vi "GetSetParam.vi"() -> ()   [LabVIEW 2020]
uses:
  lib/Snap7.lvlib
panel:
  out "?":string
  in  "Value":i64=500
  in  "Param to Set":i32(ring)=3 items=["Local Port"=1, "Remote Port"=2, "Ping Timeout (ms)"=3, "Send Timeout (ms)"=4, "Recv Timeout (ms)"=5, "Work Interval (ms)"=6, "Source REF"=7, "Destination REF"=8, "Source TSAP"=9, "PDU Request"=10, "Max Clients"=11, "BSend Timeout (ms)"=12, "BRecv Timeout (ms)"=13, "Recovery Time (ms)"=14, "Keep Alive Time (ms)"=15]
  out "ParamValue":i32
  in  "ParamNumber":i32(ring)=2 items=["Local Port"=1, "Remote Port"=2, "Ping Timeout (ms)"=3, "Send Timeout (ms)"=4, "Recv Timeout (ms)"=5, "Work Interval (ms)"=6, "Source REF"=7, "Destination REF"=8, "Source TSAP"=9, "PDU Request"=10, "Max Clients"=11, "BSend Timeout (ms)"=12, "BRecv Timeout (ms)"=13, "Recovery Time (ms)"=14, "Keep Alive Time (ms)"=15]
  out "?":string
  out "Status":string
  in  "stop":bool
  in  "Slot":i32=2
  in  "Rack":i32
  in  "Address IP":string="192.168.1.12"
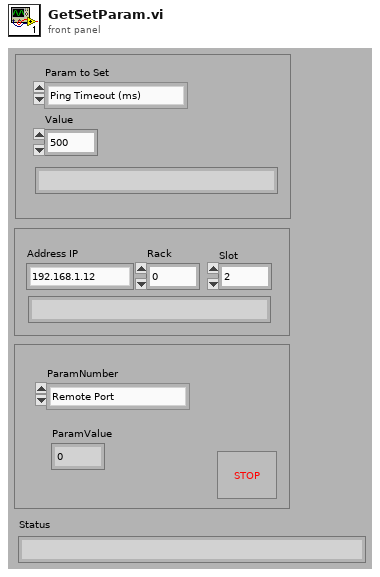
[diagram p1: front panel]
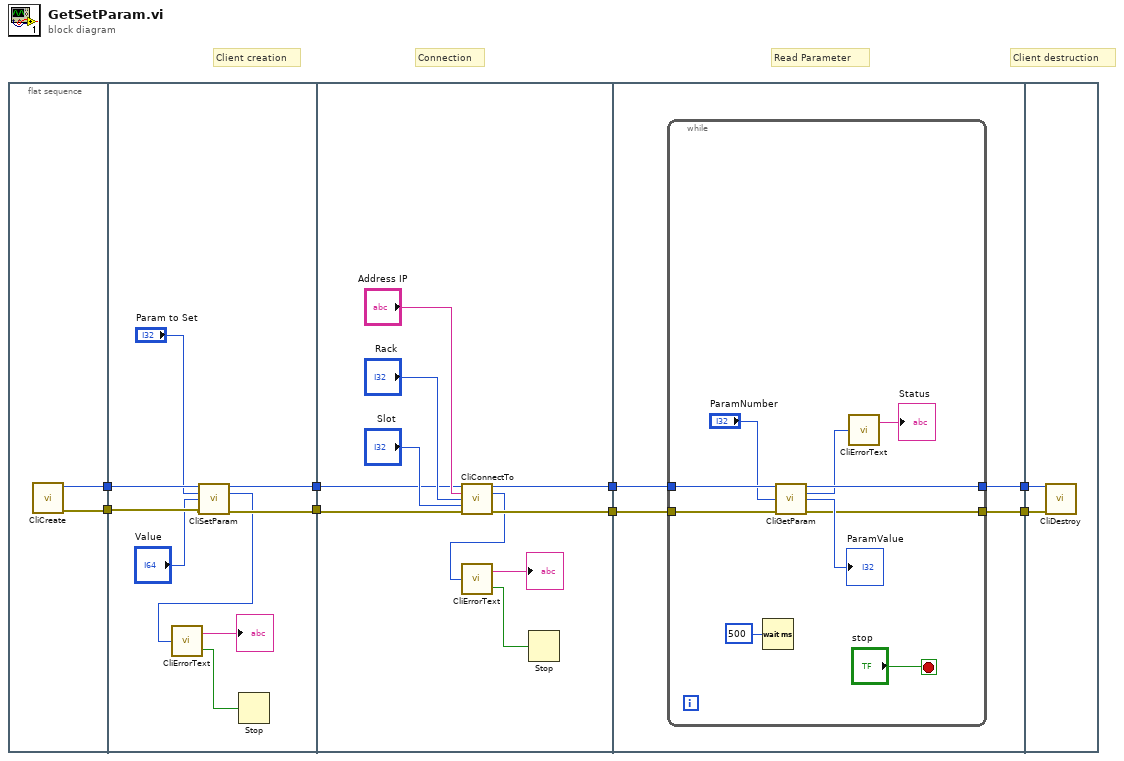
[diagram p0: block diagram]
diagram:
  # "Read Parameter"
  # "Client destruction"
  # "Connection"
  # "Client creation"
  n1 = flat-sequence {
    tunnel: [w10] -> w4
    tunnel: [w9] -> w2
    tunnel: w4 -> [w19]
    tunnel: [w18] -> w3
    tunnel: w2 -> [w17]
    tunnel: [w16] -> w1
    tunnel: [w29] -> w8
    tunnel: [w23] -> w7
    tunnel: w3 -> [w25]
    tunnel: w1 -> [w24]
    tunnel: w7 -> [w32]
    tunnel: w8 -> [w30]
    tunnel: [w33] -> w6
    tunnel: [w31] -> w5
    tunnel: w6 -> [w45]
    tunnel: w5 -> [w44]
    frame #0 {
      n2 = call "CliCreate.vi"() -> ("ref out"=w10:u64, "error out"=w9:errorcluster)  [unwired: 14 in]
    }
    frame #1 {
      n3 = call "CliSetParam.vi"("ref in"=w19, "ParamNumber"="Param to Set", "Param Value"="Value", "error in (no error)"=w17) -> ("ref out"=w18:u64, "Result"=w11:i32, "error out"=w16:errorcluster)  [unwired: 9 in]
      n4 = call "CliErrorText.vi"("ErrNo"=w11) -> ("Error"=w12:bool, "ErrMessage"=→"?":string)
      n5 = Stop(stop? (T)=w12) -> ()
    }
    frame #2 {
      n6 = call "CliConnectTo.vi"("ref in"=w25, "Address"="Address IP", "Rack"="Rack", "Slot"="Slot", "error in (no error)"=w24) -> ("ref out"=w23:u64, "Result"=w20:i32, "error out"=w29:errorcluster)  [unwired: 8 in]
      n7 = call "CliErrorText.vi"("ErrNo"=w20) -> ("Error"=w21:bool, "ErrMessage"=→"?":string)
      n8 = Stop(stop? (T)=w21) -> ()
    }
    frame #3 {
      n9 = while {
        tunnel: [w40] -> w33
        tunnel: w32 -> [w39]
        tunnel: [w38] -> w31
        tunnel: w30 -> [w37]
        stop <- "stop" stop-if-true
        n10 = Wait (ms)(milliseconds to wait=u32 500 ("Loop Delay (ms)")) -> ()  [unwired: 1 out]
        n11 = call "CliGetParam.vi"("ref in"=w39, "ParamNumber"="ParamNumber", "error in (no error)"=w37) -> ("ref out"=w40:u64, "Result"=w36:i32, "ParamValue"=→"ParamValue":i32, "error out"=w38:errorcluster)  [unwired: 9 in]
        n12 = call "CliErrorText.vi"("ErrNo"=w36) -> ("ErrMessage"=→"Status":string)  [unwired: 1 out]
      }
    }
    frame #4 {
      n13 = call "CliDestroy.vi"("ref in"=w45, "error in (no error)"=w44) -> ()  [unwired: 13 in, 1 out]
    }
  }
